vi "ziGetEventScopeWaveEX.vi"(8 "Error In":errorcluster, 11 "Handle In":T2 {"Handle" format="0x%08x"; "Conn" format="0x%08x"}) -> (0 "Error Out":errorcluster, 2 "ScopeWave Out":T1(array[cluster]), 3 "Handle Out":T2 {"Handle" format="0x%08x"; "Conn" format="0x%08x"})   [LabVIEW 2018, in "Zurich Instruments LabOne.lvlib"]
doc: "This vi retrives scope data. This function processes the data, splits the data according to the channels and incorporate the scaling / offset factor. Please, beware that in the case of HF2 a manual scaling has to be applied. Please see the ziExample-Scope.vi.The data may be formatted differently, depending on settings of the scope. See the description of the structure members for details."
uses:
  Zurich Instruments LabOne.lvlib
  ziGetEventScopeWave.vi
  ziTypeHandle.ctl
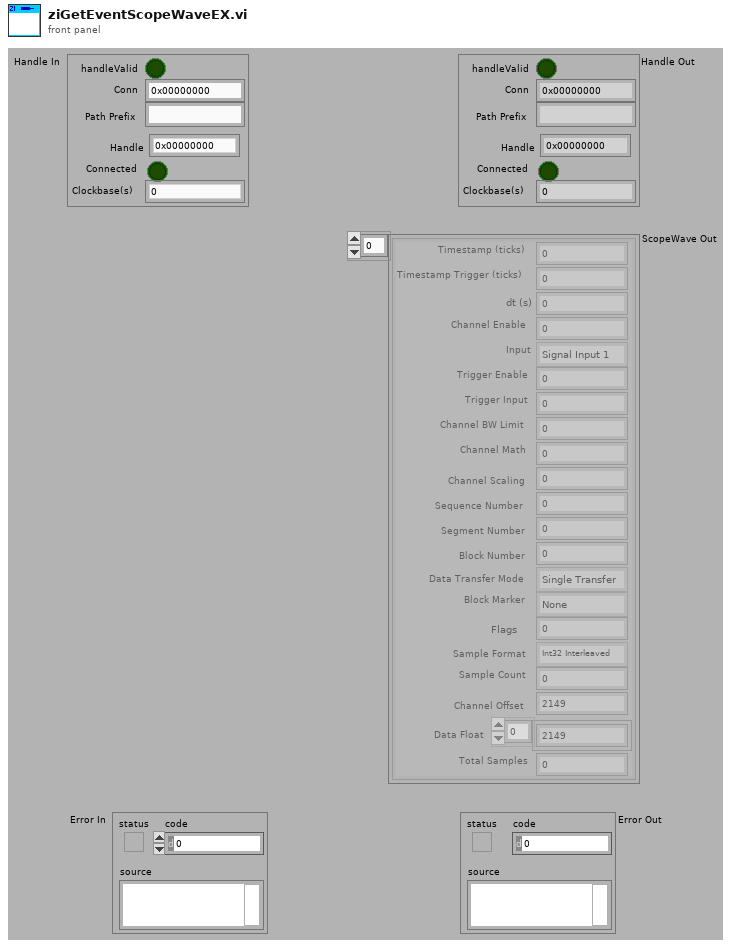
[diagram p1: front panel]
types:
  T1 = cluster{"Timestamp (ticks)":u64, "Timestamp Trigger (ticks)":u64, "dt (s)":dbl, "Channel Enable":u8, "Input":enum8{"Signal Input 1", "Signal Input 2", "Trigger Input 1", "Trigger Input 2", "Aux Output 1", "Aux Output 2", "Aux Output 3", "Aux Output 4", "Aux Input 1", "Aux Input 2"}, "Trigger Enable":u64, "Trigger Input":u64, "Channel BW Limit":u8, "Channel Math":u8, "Channel Scaling":sgl, "Sequence Number":u32, "Segment Number":u32, "Block Number":u32, "Data Transfer Mode":enum8{"Single Transfer", "Block Transfer", "Continuous Transfer", "FFT Single Transfer"}, "Block Marker":enum8{"None", "End of Block"}, "Flags":u8, "Sample Format":enum8{"Int16", "Int32", "Float32", "reserved", "Int16 Interleaved", "Int32 Interleaved", "Float32 Interleaved"}, "Sample Count":u32, "Channel Offset":dbl, "Data Float":sgl[], "Total Samples":u64}[]
  T2 = typedef "Zurich Instruments LabOne.lvlib/ziTypeHandle.ctl" = cluster{"handleValid":bool, "Conn":u64, "Path Prefix":string, "Handle":u64, "Connected":bool, "Clockbase(s)":dbl}
  T3 = typedef "Zurich Instruments LabOne.lvlib/ziTypeScopeWave.ctl" = cluster{"Timestamp (ticks)":u64, "Timestamp Trigger (ticks)":u64, "dt (s)":dbl, "Channel Enable":u8[], "Channel Input":enum8{"Signal Input 1", "Signal Input 2", "Trigger Input 1", "Trigger Input 2", "Aux Output 1", "Aux Output 2", "Aux Output 3", "Aux Output 4", "Aux Input 1", "Aux Input 2"}[], "Trigger Enable":u64, "Trigger Input":u64, "Channel BW Limit":u8[], "Channel Math":u8[], "Channel Scaling":sgl[], "Sequence Number":u32, "Segment Number":u32, "Block Number":u32, "Data Transfer Mode":enum8{"Single Transfer", "Block Transfer", "Continuous Transfer", "FFT Single Transfer"}, "Block Marker":enum8{"None", "End of Block"}, "Flags":u8, "Sample Format":enum8{"Int16", "Int32", "Float32", "reserved", "Int16 Interleaved", "Int32 Interleaved", "Float32 Interleaved"}, "Sample Count":u32, "Channel Offset":dbl[], "Data Int16":i16[], "Data Int32":i32[], "Data Float":sgl[], "Total Samples":u64}
  T4 = enum8{"Signal Input 1", "Signal Input 2", "Trigger Input 1", "Trigger Input 2", "Aux Output 1", "Aux Output 2", "Aux Output 3", "Aux Output 4", "Aux Input 1", "Aux Input 2"}[]
  T5 = enum8{"Single Transfer", "Block Transfer", "Continuous Transfer", "FFT Single Transfer"}
  T6 = enum8{"Int16", "Int32", "Float32", "reserved", "Int16 Interleaved", "Int32 Interleaved", "Float32 Interleaved"}
  T7 = cluster{"Timestamp (ticks)":u64, "Timestamp Trigger (ticks)":u64, "dt (s)":dbl, "Channel Enable":u8, "Input":enum8{"Signal Input 1", "Signal Input 2", "Trigger Input 1", "Trigger Input 2", "Aux Output 1", "Aux Output 2", "Aux Output 3", "Aux Output 4", "Aux Input 1", "Aux Input 2"}, "Trigger Enable":u64, "Trigger Input":u64, "Channel BW Limit":u8, "Channel Math":u8, "Channel Scaling":sgl, "Sequence Number":u32, "Segment Number":u32, "Block Number":u32, "Data Transfer Mode":enum8{"Single Transfer", "Block Transfer", "Continuous Transfer", "FFT Single Transfer"}, "Block Marker":enum8{"None", "End of Block"}, "Flags":u8, "Sample Format":enum8{"Int16", "Int32", "Float32", "reserved", "Int16 Interleaved", "Int32 Interleaved", "Float32 Interleaved"}, "Sample Count":u32, "Channel Offset":dbl, "Data Float":sgl[], "Total Samples":u64}
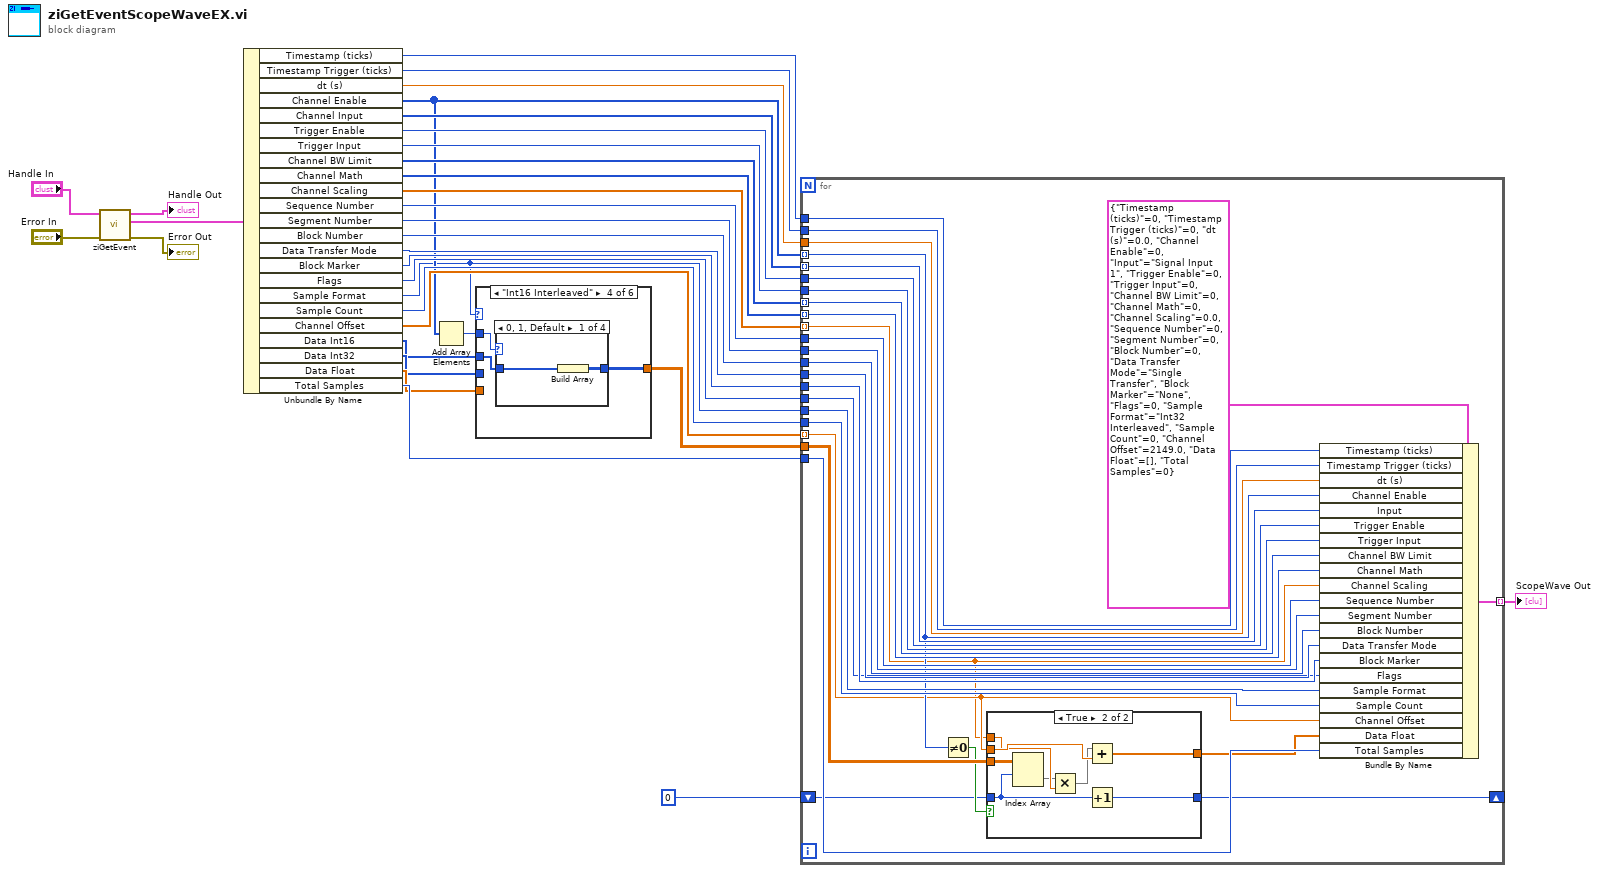
[diagram p0: block diagram]
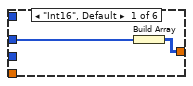
[diagram p2: hidden frame]
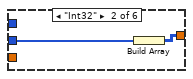
[diagram p3: hidden frame]
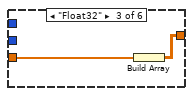
[diagram p4: hidden frame]
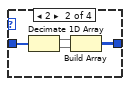
[diagram p5: hidden frame]
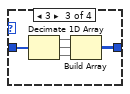
[diagram p6: hidden frame]
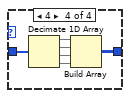
[diagram p7: hidden frame]
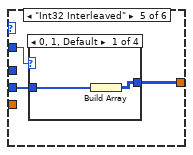
[diagram p8: hidden frame]
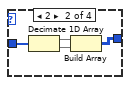
[diagram p9: hidden frame]
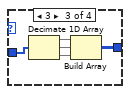
[diagram p10: hidden frame]
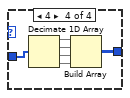
[diagram p11: hidden frame]
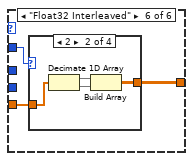
[diagram p12: hidden frame]
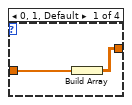
[diagram p13: hidden frame]
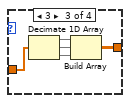
[diagram p14: hidden frame]
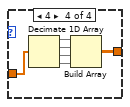
[diagram p15: hidden frame]
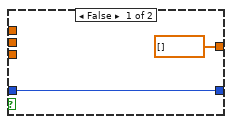
[diagram p16: hidden frame]
diagram:
  n1 = call-poly "ziGetEvent.vi"("Error In"="Error In", "Handle In"="Handle In") -> ("Error Out"=→"Error Out":errorcluster, "ScopeWave Out"=w12:T3, "Handle Out"=→"Handle Out":T2)  [unwired: 7 in]
  n2 = Unbundle By Name(w12) -> ("Timestamp (ticks)"=w30:u64, "Timestamp Trigger (ticks)"=w29:u64, "dt (s)"=w11:dbl, "Channel Enable"=w7:u8[], "Channel Input"=w28:T4, "Trigger Enable"=w27:u64, "Trigger Input"=w26:u64, "Channel BW Limit"=w25:u8[], "Channel Math"=w24:u8[], "Channel Scaling"=w23:sgl[], "Sequence Number"=w22:u32, "Segment Number"=w21:u32, "Block Number"=w20:u32, "Data Transfer Mode"=w19:T5, "Block Marker"=w18:enum8{"None", "End of Block"}, "Flags"=w17:u8, "Sample Format"=w1:T6, "Sample Count"=w16:u32, "Channel Offset"=w15:dbl[], "Data Int16"=w8:i16[], "Data Int32"=w9:i32[], "Data Float"=w10:sgl[], "Total Samples"=w14:u64)
  n3 = Add Array Elements(numeric array=w7) -> (sum=w6:u8)
  n4 = case shown="\"Int16 Interleaved\"" w1 {
    tunnel: [w34 w36 w38 w41 w61 w80] -> w5
    tunnel: w10 -> [_ _ w37 _ _ w81]
    tunnel: w8 -> [w33 _ _ w40 _ _]
    tunnel: w9 -> [_ w35 _ _ w60 _]
    tunnel: w6 -> [_ _ _ w39 w59 w79]
    frame "Int16", Default {
      n5 = Build Array(w33) -> (w34:i16[][])
    }
    frame "Int32" {
      n6 = Build Array(w35) -> (w36:i32[][])
    }
    frame "Float32" {
      n7 = Build Array(w37) -> (w38:sgl[][])
    }
    frame "Int16 Interleaved" {
      n8 = case shown="0, 1, Default" w39 {
        tunnel: w40 -> [w43 w47 w52 w58]
        tunnel: [w42 w46 w51 w57] -> w41
        frame 0, 1, Default {
          n9 = Build Array(w43) -> (w42:i16[][])
        }
        frame 2 {
          n10 = Decimate 1D Array(w47) -> (w45:i16[], w44:i16[])
          n11 = Build Array(w45, w44) -> (w46:i16[][])
        }
        frame 3 {
          n12 = Decimate 1D Array(w52) -> (w50:i16[], w49:i16[], w48:i16[])
          n13 = Build Array(w50, w49, w48) -> (w51:i16[][])
        }
        frame 4 {
          n14 = Decimate 1D Array(w58) -> (w56:i16[], w55:i16[], w54:i16[], w53:i16[])
          n15 = Build Array(w56, w55, w54, w53) -> (w57:i16[][])
        }
      }
    }
    frame "Int32 Interleaved" {
      n16 = case shown="0, 1, Default" w59 {
        tunnel: w60 -> [w63 w67 w72 w78]
        tunnel: [w62 w66 w71 w77] -> w61
        frame 0, 1, Default {
          n17 = Build Array(w63) -> (w62:i32[][])
        }
        frame 2 {
          n18 = Decimate 1D Array(w67) -> (w65:i32[], w64:i32[])
          n19 = Build Array(w65, w64) -> (w66:i32[][])
        }
        frame 3 {
          n20 = Decimate 1D Array(w72) -> (w70:i32[], w69:i32[], w68:i32[])
          n21 = Build Array(w70, w69, w68) -> (w71:i32[][])
        }
        frame 4 {
          n22 = Decimate 1D Array(w78) -> (w76:i32[], w75:i32[], w74:i32[], w73:i32[])
          n23 = Build Array(w76, w75, w74, w73) -> (w77:i32[][])
        }
      }
    }
    frame "Float32 Interleaved" {
      n24 = case shown="2" w79 {
        tunnel: w81 -> [w83 w87 w92 w98]
        tunnel: [w82 w86 w91 w97] -> w80
        frame 0, 1, Default {
          n25 = Build Array(w83) -> (w82:sgl[][])
        }
        frame 2 {
          n26 = Decimate 1D Array(w87) -> (w85:sgl[], w84:sgl[])
          n27 = Build Array(w85, w84) -> (w86:sgl[][])
        }
        frame 3 {
          n28 = Decimate 1D Array(w92) -> (w90:sgl[], w89:sgl[], w88:sgl[])
          n29 = Build Array(w90, w89, w88) -> (w91:sgl[][])
        }
        frame 4 {
          n30 = Decimate 1D Array(w98) -> (w96:sgl[], w95:sgl[], w94:sgl[], w93:sgl[])
          n31 = Build Array(w96, w95, w94, w93) -> (w97:sgl[][])
        }
      }
    }
  }
  n32 = for {
    tunnel: w30 -> [w124]
    tunnel: w29 -> [w123]
    tunnel: w7 -> [w104] mode=indexing
    tunnel: w28 -> [w108] mode=indexing
    tunnel: w27 -> [w113]
    tunnel: w26 -> [w112]
    tunnel: w25 -> [w111] mode=indexing
    tunnel: w24 -> [w110] mode=indexing
    tunnel: w23 -> [w102] mode=indexing
    tunnel: w22 -> [w121]
    tunnel: w21 -> [w120]
    tunnel: w20 -> [w119]
    tunnel: w19 -> [w118]
    tunnel: w18 -> [w117]
    tunnel: w17 -> [w116]
    tunnel: w1 -> [w107]
    tunnel: w16 -> [w115]
    tunnel: w15 -> [w103] mode=indexing
    tunnel: w14 -> [w114]
    tunnel: [w125] -> w13 mode=indexing
    tunnel: w11 -> [w109]
    tunnel: w5 -> [w106]
    shift-right: [w100] -> _
    shift-left: 0 -> [w99]
    n33 = Not Equal To 0?(x=w104) -> (x != 0?=w105:bool)
    n34 = case shown="True" w105 {
      tunnel: w106 -> [_ w135]
      tunnel: w99 -> [w126 w129]
      tunnel: w103 -> [_ w134]
      tunnel: w102 -> [_ w132]
      tunnel: [dbl[] [] w130] -> w101
      tunnel: [w126 w128] -> w100
      frame False {
      }
      frame True {
        n35 = Index Array(array=w135, index (row)=w129) -> (element=w131:sgl[])  [unwired: 1 in]
        n36 = Multiply(x=w131, y=w132) -> (x*y=w133:sgl[])
        n37 = Add(x=w133, y=w134) -> (x+y=w130:dbl[])
        n38 = Increment(x=w129) -> (x+1=w128:i32)
      }
    }
    n39 = Bundle By Name(cluster=T7 {"Timestamp (ticks)"=0, "Timestamp Trigger (ticks)"=0, "dt (s)"=0.0, "Channel Enable"=0, "Input"=enum."Signal Input 1", "Trigger Enable"=0, "Trigger Input"=0, "Channel BW Limit"=0, "Channel Math"=0, "Channel Scaling"=0.0, "Sequence Number"=0, "Segment Number"=0, "Block Number"=0, "Data Transfer Mode"=enum."Single Transfer", "Block Marker"=enum."None", "Flags"=0, "Sample Format"=enum."Int32 Interleaved", "Sample Count"=0, "Channel Offset"=2149.0, "Data Float"=[], "Total Samples"=0} ("ScopeWave Out 2"), "Timestamp (ticks)"=w124, "Timestamp Trigger (ticks)"=w123, "dt (s)"=w109, "Channel Enable"=w104, "Input"=w108, "Trigger Enable"=w113, "Trigger Input"=w112, "Channel BW Limit"=w111, "Channel Math"=w110, "Channel Scaling"=w102, "Sequence Number"=w121, "Segment Number"=w120, "Block Number"=w119, "Data Transfer Mode"=w118, "Block Marker"=w117, "Flags"=w116, "Sample Format"=w107, "Sample Count"=w115, "Channel Offset"=w103, "Data Float"=w101, "Total Samples"=w114) -> (w125:T7)
  }
  "ScopeWave Out" <- w13
